vi "Read Matlab Params.vi"(8 "error in (no error)":errorcluster, 10 "Enum":enum16{"StartSession", "StartTrial"}(ring), 11 "TrialBasedExperiment in":refnum<class "BehaviorClassification.lvclass">) -> (0 "error out":errorcluster, 2 "Matlab Param Array":cluster{"Name":string, "Data":variant}[](array[cluster]), 3 "TrialBasedExperiment out":refnum<class "BehaviorClassification.lvclass">)   [LabVIEW 2010, in "BehaviorClassification.lvclass"]
uses:
  BehaviorClassification.lvclass
  MatlabExperiment/MatlabExperiment.lvclass
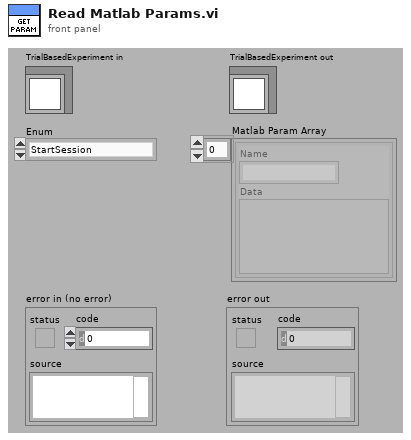
[diagram p1: front panel]
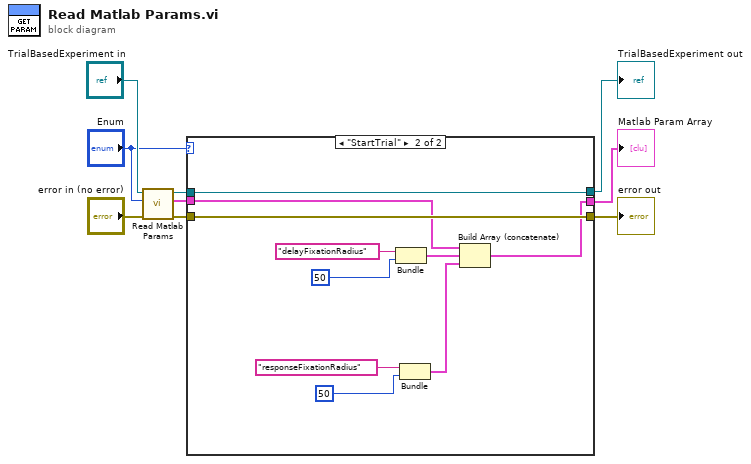
[diagram p0: block diagram]
diagram:
  n1 = call-parent "Read Matlab Params.vi"("error in (no error)"="error in (no error)", "Enum"="Enum", "TrialBasedExperiment in"="TrialBasedExperiment in") -> ("error out"=w5:errorcluster, "Matlab Param Array"=w4:cluster{"Name":string, "Data":variant}[], "TrialBasedExperiment out"=w6:refnum<class "BehaviorClassification.lvclass">)  [unwired: 6 in]
  n2 = case shown="\"StartTrial\"" "Enum" {
    tunnel: w6 -> [w12 w22]
    tunnel: w5 -> [w11 w21]
    tunnel: [w12 w22] -> w2
    tunnel: w4 -> [w10 w18]
    tunnel: [w11 w21] -> w3
    tunnel: [w10 w16] -> w1
    frame "StartSession", Default {
    }
    frame "StartTrial" {
      n3 = Bundle("delayFixationRadius", 50) -> (w17:cluster{string, i32})  [unwired: 1 out]
      n4 = Bundle("responseFixationRadius", 50) -> (w13:cluster{string, i32})  [unwired: 1 out]
      n5 = Build Array (concatenate)(w18, w17, w13) -> (w16:cluster{"Name":string, "Data":variant}[])
    }
  }
  "error out" <- w3
  "TrialBasedExperiment out" <- w2
  "Matlab Param Array" <- w1
